vi "Write.Data.Buffer.vi"(8 "error in":errorcluster, 9 "Offset":i32, 10 "Values":dbl[](array[numeric]), 11 "Ref":T1) -> (0 "error out":errorcluster)   [LabVIEW 2027, in "Data Access Engine (Express).lvlib" / "Data Access Engine (Express).lvclass"]
uses:
  Data Access Engine (Express).lvclass
  Types/Write.DVR.ctl
  Access Type Classes/Write/Write.lvclass
  Access Type Classes/Write/Write.lvclass/Write.ctl
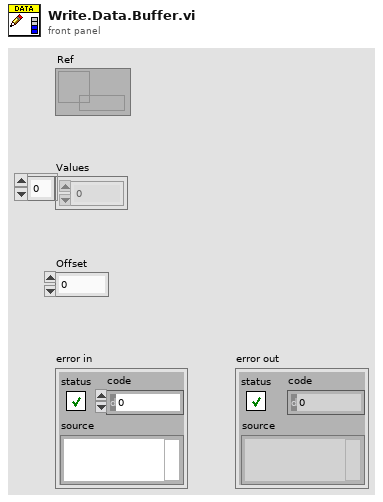
[diagram p1: front panel]
types:
  T1 = typedef "Data Access Engine (Express).lvlib/Data Access Engine (Express).lvclass/Write.DVR.ctl" = refnum<data-value>
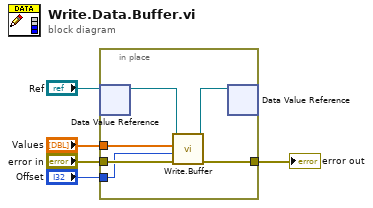
[diagram p0: block diagram]
diagram:
  n1 = in-place {
    in-place-border: "error in" -> [w11]
    in-place-border: [w10] -> w4
    in-place-border: "Values" -> [w7]
    in-place-border: "Offset" -> [w6]
    n2 = in-place-dvr #1("Ref") -> (w9:refnum<class "Write.lvclass">)  [unwired: 1 out]
    n3 = call "Write.Buffer.vi"("error in"=w11, "Offset"=w6, "Values"=w7, "Write in"=w9) -> ("error out"=w10:errorcluster, "Write out"=w8:refnum<class "Write.lvclass">)  [unwired: 6 in]
    n4 = in-place-dvr #1(w8) -> ()  [unwired: 2 out]
  }
  "error out" <- w4
